vi "Initialize.vi"(8 "error in":errorcluster, 9 "Channels Amount":u8=1, 10 "InstanceName":string, 11 "Device Cluster.lvclass":refnum<class "Device Cluster.lvclass">) -> (0 "error out":errorcluster, 3 "Device Cluster.lvclass out":refnum<class "Device Cluster.lvclass">)   [LabVIEW 2023, in "Device Cluster.lvclass"]
uses:
  Device Cluster.lvclass
  Device Cluster.lvclass/Device Cluster.ctl
  78d7c854-17cb-40e3-91c7-b55f38b06fec.vi
  34d8de8f-da75-496c-99f7-44cc67c60a3e.vi
  78d7c854-17cb-40e3-91c7-b55f38b06fec.vi/4bc1c15b-36ab-481f-b8dd-c64075ce723a.vi
  34d8de8f-da75-496c-99f7-44cc67c60a3e.vi/4bc1c15b-36ab-481f-b8dd-c64075ce723a.vi
  <vilib>/ADAS Replay HIL/AdasHilServices/AdasHilServices Fill In Error Info Ex.vi
  Utilities/Utilities.lvlib
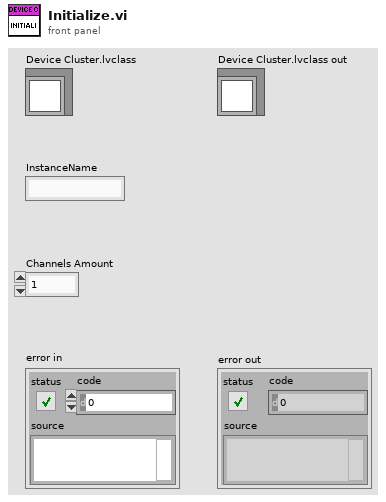
[diagram p1: front panel]
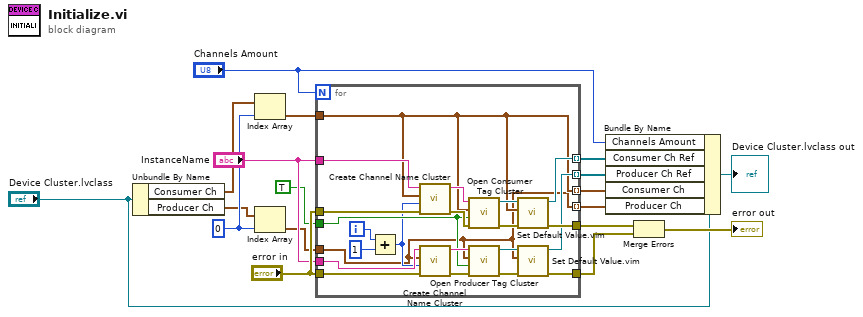
[diagram p0: block diagram]
diagram:
  w5 = 0 ("index")
  n1 = Unbundle By Name("Device Cluster.lvclass") -> ("Consumer Ch"=w7:cluster{"Voltage.SP":dbl, "Current.SP":dbl}[], "Producer Ch"=w4:cluster{"Voltage.AV":dbl, "Current.AV":dbl}[])
  n2 = Index Array(array=w7, index=w5) -> (element=w6:cluster{"Voltage.SP":dbl, "Current.SP":dbl})
  n3 = Index Array(array=w4, index=w5) -> (element=w3:cluster{"Voltage.AV":dbl, "Current.AV":dbl})
  n4 = for {
    N: "Channels Amount" -> [_]
    tunnel: "error in" -> [w32]
    tunnel: "InstanceName" -> [w31]
    tunnel: "error in" -> [w30]
    tunnel: "InstanceName" -> [w29]
    tunnel: [w28] -> w15
    tunnel: [w27] -> w14
    tunnel: [w26] -> w12 mode=indexing
    tunnel: [w25] -> w11 mode=indexing
    tunnel: w6 -> [w20]
    tunnel: w3 -> [w19]
    tunnel: TRUE ("Create if not found? (T)") -> [w24]
    tunnel: [w20] -> w2 mode=indexing
    tunnel: [w19] -> w1 mode=indexing
    i -> [w23]
    n5 = Add(x=w23, y=1) -> (x+y=w22:i32)
    n6 = call "Create Channel Name Cluster.vi"("error in"=w30, "Numeric"=w22, "Cluster"=w20, "Instance Name"=w29) -> ("error out"=w38:errorcluster, "Data Channel Name"=w33:string)  [unwired: 6 in]
    n7 = call "Create Channel Name Cluster.vi"("error in"=w32, "Numeric"=w22, "Cluster"=w19, "Instance Name"=w31) -> ("error out"=w40:errorcluster, "Data Channel Name"=w34:string)  [unwired: 6 in]
    n8 = call "Open Consumer Tag Cluster.vi"("error in"=w38, "Create if not found? (T)"=w24, "Cluster"=w20, "Channel Name"=w33) -> ("error out"=w37:errorcluster, "ADAS HIL Channel"=w36:refnum<k21>)  [unwired: 6 in]
    n9 = call "Open Producer Tag Cluster.vi"("error in"=w40, "Create if not found? (T)"=w24, "Cluster"=w19, "Channel Name"=w34) -> ("error out"=w39:errorcluster, "ADAS HIL Channel"=w35:refnum<k21>)  [unwired: 6 in]
    n10 = call "Set Default Value.vim"("error in"=w37, "Data in"=w20, "ADAS HIL Channel in"=w36) -> ("error out"=w27:errorcluster, "ADAS HIL Channel out"=w26:refnum<k21>)  [unwired: 7 in]
    n11 = call "Set Default Value.vim"("error in"=w39, "Data in"=w19, "ADAS HIL Channel in"=w35) -> ("error out"=w28:errorcluster, "ADAS HIL Channel out"=w25:refnum<k21>)  [unwired: 7 in]
  }
  n12 = Bundle By Name(cluster="Device Cluster.lvclass", "Channels Amount"="Channels Amount", "Consumer Ch Ref"=w12, "Producer Ch Ref"=w11, "Consumer Ch"=w2, "Producer Ch"=w1) -> (→"Device Cluster.lvclass out":refnum<class "Device Cluster.lvclass">)
  n13 = Merge Errors(w14, w15) -> (→"error out":errorcluster)
